vi "Resolve Missing Dependency - Custom gRPC Service Core.vi"(8 "error in":errorcluster, 10 "Project Name":string, 11 "Map - LibRef":map{string, refnum<vi>}(c390)) -> (0 "error out":errorcluster)   [LabVIEW 2023, in "Plugin Generator.lvlib"]
uses:
  Plugin Generator.lvlib
  <vilib>/dlg_ctls.llb/Space Constant.vi
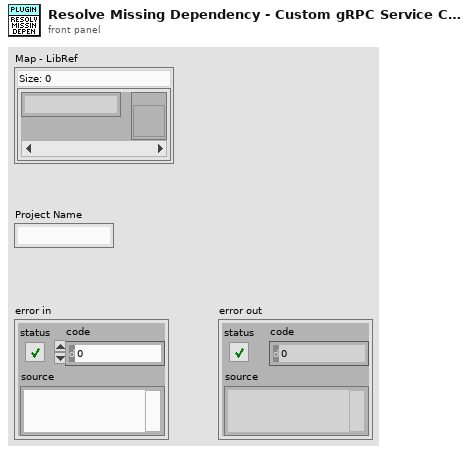
[diagram p1: front panel]
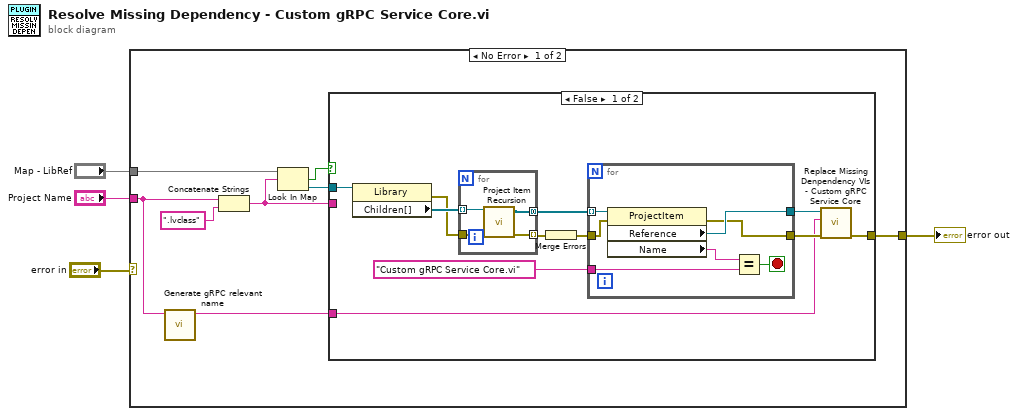
[diagram p0: block diagram]
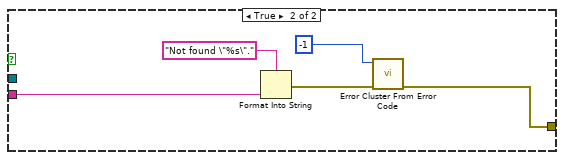
[diagram p2: hidden frame]
diagram:
  n1 = case shown="No Error" "error in" {
    selector: "error in" -> [_ w40]
    tunnel: [w12 w40] -> w4
    tunnel: "Map - LibRef" -> [w8 _]
    tunnel: "Project Name" -> [w7 _]
    frame No Error {
      n2 = call "Generate gRPC relevant name.vi"("Project Name"=w7) -> ("gRPC Service Name"=w6:string)  [unwired: 9 in, 1 out]
      n3 = Concatenate Strings(w7, ".lvclass" ("String")) -> (w5:string)
      n4 = Look In Map(map=w8, key=w5) -> (key not found?=w10:bool, value=w11:refnum<vi>)  [unwired: 1 in]
      n5 = case shown="False" w10 {
        tunnel: w11 -> [w23 _]
        tunnel: [w16 w36] -> w12
        tunnel: w6 -> [w15 _]
        tunnel: w5 -> [_ w35]
        frame False {
          n6 = property class="Library"(reference=w23) -> (error out=w21:errorcluster, "Children[]"=w22:refnum<vi>[])  [unwired: 1 in, 1 out]
          n7 = for {
            tunnel: w22 -> [w34] mode=indexing
            tunnel: [w33] -> w20 mode=concatenating
            tunnel: w21 -> [w32]
            tunnel: [w31] -> w13 mode=indexing
            n8 = call "Project Item Recursion.vi"("error in"=w32, "TargetItem in"=w34) -> ("error out"=w31:errorcluster, "TargetItem out"=w33:refnum<vi>[])  [unwired: 8 in]
          }
          n9 = Merge Errors(w13) -> (w14:errorcluster)
          n10 = for {
            tunnel: w20 -> [w30] mode=indexing
            tunnel: "Custom gRPC Service Core.vi" ("String") -> [w28]
            tunnel: [w26] -> w18
            tunnel: [w25] -> w17
            tunnel: w14 -> [w24]
            stop <- w29 stop-if-true
            n11 = property class="ProjectItem"(reference=w30, error in=w24) -> (error out=w25:errorcluster, "Reference"=w26:refnum<vi>, "Name"=w27:string)  [unwired: 1 out]
            n12 = Equal?(x=w27, y=w28) -> (x = y?=w29:bool)
          }
          n13 = call "Replace Missing Denpendency VIs - Custom gRPC Service Core.vi"("error in"=w17, "gRPC Service Name"=w15, "VI Refnum"=w18) -> ("error out"=w16:errorcluster)  [unwired: 8 in]
        }
        frame True {
          n14 = Format Into String(format string="Not found \"%s\"." ("error message (\"\")"), w35) -> (error out=w38:errorcluster)  [unwired: 2 in, 1 out]
          n15 = call <vilib>:"Error Cluster From Error Code.vi"("error in (no error)"=w38, "error code (0)"=-1) -> ("error out"=w36:errorcluster)  [unwired: 7 in]
        }
      }
    }
    frame Error {
    }
  }
  "error out" <- w4
